vi "Test3-v3-copy1.vi"() -> ()   [LabVIEW 2023]
uses:
  <vilib>/Analysis/8numeric.llb/1D Numeric Integration.vi
  <vilib>/Analysis/NI_AALPro.lvlib
panel:
  out "Is XMotion Done":bool
  out "millisecond timer value":u32
  in  "DoNOT USE":bool
  out "subarray":i32[](array[numeric])
  out "Number areas":i32=1
  out "Gain description":string[](array[string])
  out "ADC description":string[](array[string])
  out "Gain Number":i32[](array[numeric])
  out "activeYPixels":i32=256
  out "activeXPixels":i32=1024
  out "Is YMotion Done":bool
  out "error out":errorcluster
  out "Identification":string
  out "DeviceKey Out":string
  out "Filename":path caption="Filename Out"
  in  "Save?":bool=TRUE caption="Enable"
  in  "CCD Busy 2":bool caption="CCD Busy"
  in  "stop":bool
  in  "Start Scan":bool caption="Acquire"
  out "Acq Time(ms)":u32
  in  "ShutterOpen":bool
  in  "DisplayArea":i32
  in  "numAreas":i32=2
  out "Gain_supplied":i32
  out "ADC_supplied":i32
  out "DataSize":i32
  in  "Number of Areas :":u16=1 min=1 step=1
  in  "Integration time (ms)":i16
  out "ADC Number":i32[](array[numeric])
  out "FirmwareVersion":string="V1.89  CCD_3000"
  out "nbr of components":i32
  out "CCD DeviceName":string[](array[string])
  out "CCD UniqueID":string[](array[string])
  out "Xloop_iter":i32
  out "Yloop_iter":i32
  out "YPos":i32
  out "XPos":i32
  in  "Xtotalsteps":i32
  in  "Xstep_res (BWD)":i32
  in  "Xstep_res (FWD)":i32
  in  "MotorX":i32
  in  "Wait time (ms) in X":u32
  in  "MotorY":i32
  in  "Ystep_res":i32
  in  "Ytotalsteps":i32
  out "max value":i32
  in  "MinZ":dbl
  in  "StopIn":dbl
  in  "StartIn":i32
  out "AreaUnder":dbl format="%0.4f"
  out "Intensity Graph":dbl[][](graph)=[[0.0, 960.0, 940.0, 790.0, 950.0, 1030.0, 970.0, 780.0, 990.0, 1010.0, 980.0, 900.0, 1080.0, 950.0, 890.0, 1020.0, 780.0, 1020.0, 950.0, 1180.0], [800.0, 720.0, 880.0, 950.0, 850.0, 960.0, 940.0, 970.0, 830.0, 1050.0, 1140.0, 870.0, 1000.0, 1340.0, 860.0, 1760.0, 980.0, 1900.0, 1120.0, 1650.0], [770.0, 1000.0, 1080.0, 820.0, 880.0, 880.0, 1170.0, 900.0, 750.0, 1110.0, 950.0, 820.0, 780.0, 1510.0, 710.0, 3630.0, 770.0, 4530.0, 1060.0, 4960.0], [570.0, 1040.0, 990.0, 1300.0, 770.0, 940.0, 940.0, 920.0, 1010.0, 920.0, 1030.0, 1170.0, 670.0, 3990.0, 1270.0, 7770.0, 1780.0, 10190.0, 1940.0, 10320.0], [700.0, 2170.0, 720.0, 1070.0, 920.0, 1100.0, 1070.0, 1240.0, 1090.0, 1090.0, 780.0, 2330.0, 1100.0, 9500.0, 2570.0, 13250.0, 3430.0, 18370.0, 4920.0, 15420.0], [1150.0, 4050.0, 870.0, 1990.0, 990.0, 2300.0, 890.0, 2100.0, 890.0, 2030.0, 850.0, 5530.0, 1660.0, 16900.0, 6920.0, 20860.0, 8010.0, 26820.0, 11920.0, 24090.0], [2410.0, 7690.0, 1380.0, 5680.0, 950.0, 5660.0, 1150.0, 6030.0, 1120.0, 5990.0, 1100.0, 13320.0, 4680.0, 23310.0, 12680.0, 30260.0, 15460.0, 37490.0, 20040.0, 32360.0], [3730.0, 11670.0, 3470.0, 10700.0, 2160.0, 11620.0, 2650.0, 13450.0, 1960.0, 16280.0, 3330.0, 24280.0, 9750.0, 29590.0, 19490.0, 39280.0, 25460.0, 44560.0, 28710.0, 38240.0], [5820.0, 13930.0, 7980.0, 15370.0, 5380.0, 18180.0, 6410.0, 22810.0, 6360.0, 28160.0, 9770.0, 34440.0, 18410.0, 42010.0, 27930.0, 47640.0, 36930.0, 51850.0, 36620.0, 38310.0], [10910.0, 18840.0, 11150.0, 20990.0, 10890.0, 24120.0, 12390.0, 32770.0, 15080.0, 36680.0, 20580.0, 46100.0, 28750.0, 52000.0, 34670.0, 57560.0, 43850.0, 55160.0, 43260.0, 39980.0], [15940.0, 18620.0, 14810.0, 27550.0, 16710.0, 32360.0, 19800.0, 43300.0, 25930.0, 49500.0, 33140.0, 57890.0, 36190.0, 59830.0, 45190.0, 66030.0, 50740.0, 62090.0, 48710.0, 40450.0], [18210.0, 21400.0, 20610.0, 32540.0, 22470.0, 41180.0, 26870.0, 55110.0, 36190.0, 59600.0, 45000.0, 71170.0, 49620.0, 77020.0, 54950.0, 77120.0, 60070.0, 65320.0, 47310.0, 41610.0], [19980.0, 27630.0, 24900.0, 39620.0, 30920.0, 51640.0, 41210.0, 64930.0, 48560.0, 75980.0, 58830.0, 80180.0, 62620.0, 87370.0, 65050.0, 89380.0, 67340.0, 71060.0, 52720.0, 42330.0], [22060.0, 37480.0, 29730.0, 46150.0, 36490.0, 61910.0, 51530.0, 75500.0, 57820.0, 89350.0, 70600.0, 94390.0, 78340.0, 96990.0, 80350.0, 100080.0, 79370.0, 79130.0, 55810.0, 45520.0], [30290.0, 47190.0, 34090.0, 53020.0, 45160.0, 73900.0, 63850.0, 88890.0, 70560.0, 101120.0, 83090.0, 103760.0, 86430.0, 106600.0, 95730.0, 104970.0, 86060.0, 78120.0, 60830.0, 48710.0], [38810.0, 59500.0, 41970.0, 66520.0, 54310.0, 87210.0, 76860.0, 101460.0, 84910.0, 110370.0, 96060.0, 118150.0, 97970.0, 118660.0, 105500.0, 102890.0, 92680.0, 80660.0, 66370.0, 49220.0], [44290.0, 65130.0, 55290.0, 74890.0, 65450.0, 93890.0, 85000.0, 113550.0, 95920.0, 123970.0, 110280.0, 127190.0, 107900.0, 124790.0, 109070.0, 100530.0, 93780.0, 73700.0, 66770.0, 49400.0], [55930.0, 72390.0, 63110.0, 87710.0, 79530.0, 109270.0, 102450.0, 128690.0, 113170.0, 131910.0, 117470.0, 139240.0, 122700.0, 128430.0, 115300.0, 94570.0, 90710.0, 67040.0, 64120.0, 46810.0], [68310.0, 81060.0, 70150.0, 94040.0, 87080.0, 115930.0, 110550.0, 136550.0, 122470.0, 143100.0, 130550.0, 141520.0, 133000.0, 121900.0, 118010.0, 88120.0, 91940.0, 60980.0, 61360.0, 41230.0], [76260.0, 81810.0, 83610.0, 90390.0, 95690.0, 107610.0, 122620.0, 130470.0, 133680.0, 139910.0, 142260.0, 148030.0, 139440.0, 133350.0, 117890.0, 103760.0, 83410.0, 75650.0, 56860.0, 51030.0]]
  out "Data":i32[][](graph)
  out "XY Graph":cluster{"X":dbl[], "Y":dbl[]}[](graph)
  out "result":dbl format="%0.4f"
  out "areas :":i32[][](array[numeric])=[[1], [1], [1], [1440], [1032], [1], [1032]]
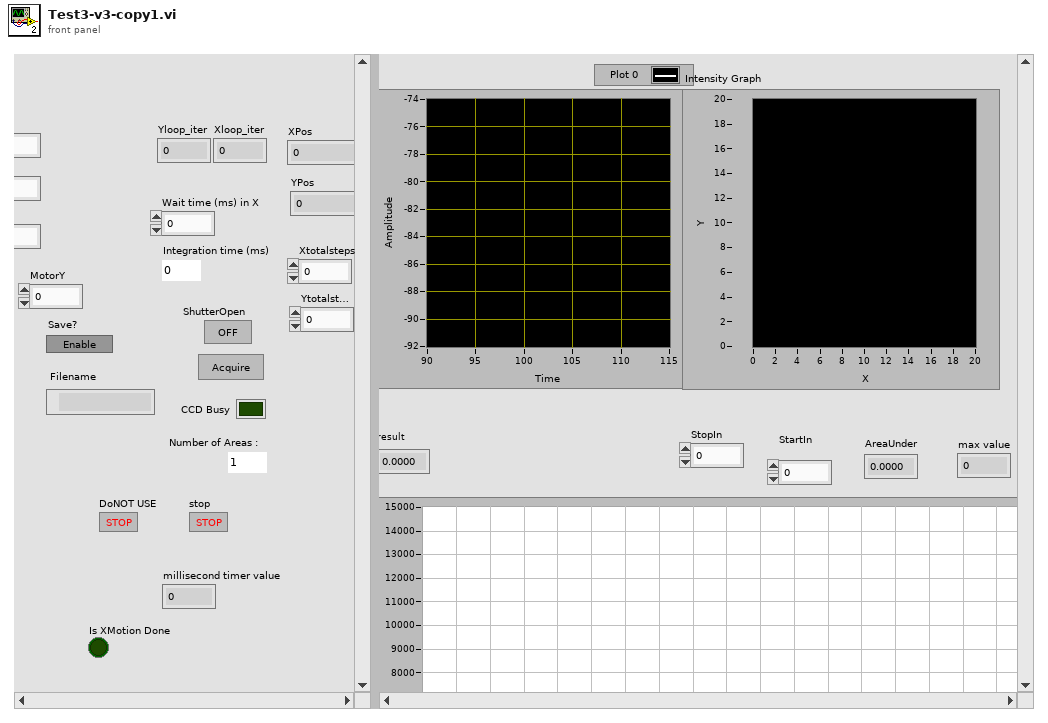
[diagram p1: front panel]
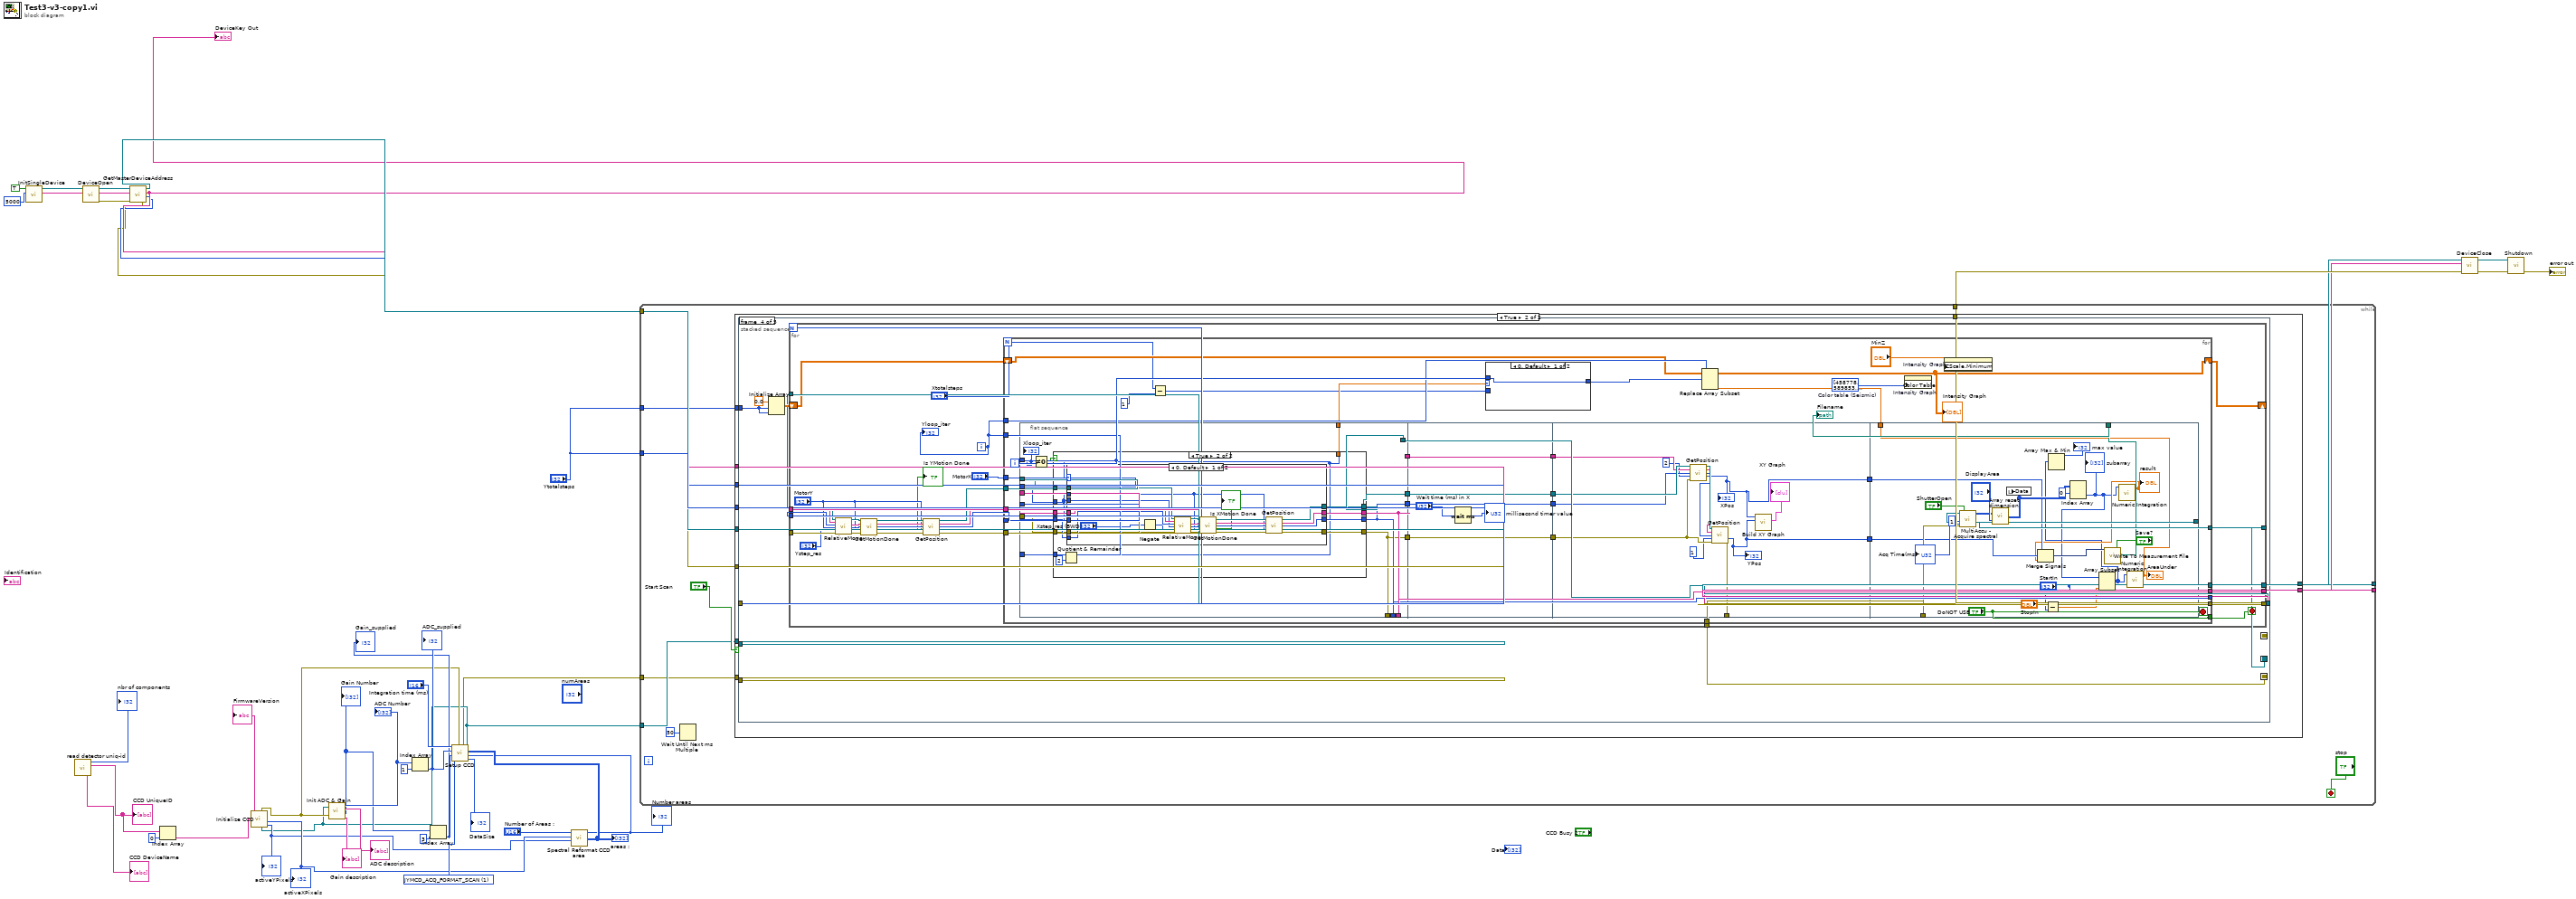
[diagram p0: block diagram]
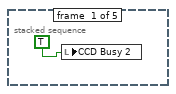
[diagram p3: hidden frame]
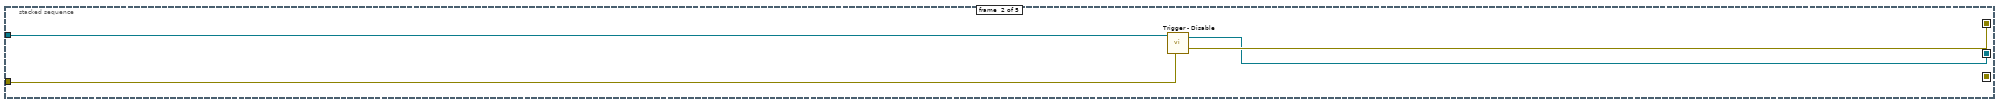
[diagram p4: hidden frame]
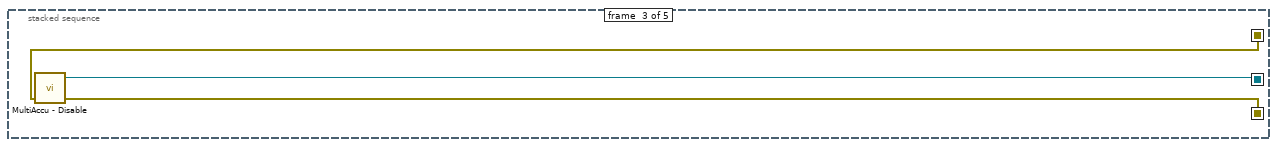
[diagram p5: hidden frame]
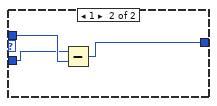
[diagram p6: hidden frame]
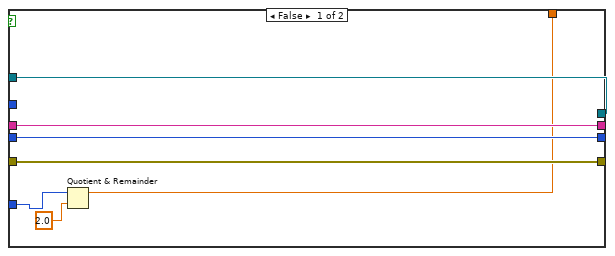
[diagram p7: hidden frame]
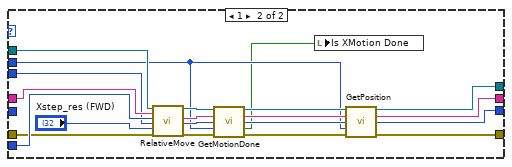
[diagram p8: hidden frame]
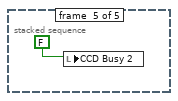
[diagram p9: hidden frame]
diagram:
  w19 = 1 items=["JYMCD_ACQ_FORMAT_IMAGE", "JYMCD_ACQ_FORMAT_SCAN"] ("Acquisition type")
  n1 = call "InitSingleDevice.vi"("msecDelayForDiscovery"=5000, "logging"=TRUE) -> ("DeviceKey Out"=w38:string, "CmdLib Out"=w39:refnum<k24>)  [unwired: 3 in, 1 out]
  n2 = call "read detector uniq-id.vi"() -> ("nbr of components"=→"nbr of components":i32, "UniqueID"=w32:string[], "DeviceName"=→"CCD DeviceName":string[])  [unwired: 3 in, 1 out]
  "CCD UniqueID" <- w32
  n3 = call "DeviceOpen.vi"("DeviceKey In"=w38, "CmdLib In"=w39) -> ("error out"=w42:errorcluster, "DeviceKey Out"=w41:string, "CmdLib Out"=w40:refnum<k24>)  [unwired: 3 in]
  n4 = call "GetMasterDeviceAddress.vi"("error in (no error)"=w42, "DeviceKey In"=w41, "CmdLib In"=w40) -> ("error out"=w5:errorcluster, "Device Address"=w6:i32, "DeviceKey Out"=w7:string, "CmdLib Out"=w8:refnum<k24>)  [unwired: 1 in]
  "DeviceKey Out" <- w7
  n5 = Index Array(array=w32, index=0) -> (element=w30:string)
  n6 = call "Initialize CCD.vi"("Unique id:"=w30) -> ("activeYPixels"=w16:i32, "JYCCDLib.IJYCCDReqd"=w10:refnum<k7>, "activeXPixels"=w17:i32, "sortie d'erreur"=w18:errorcluster, "FirmwareVersion"=→"FirmwareVersion":string)  [unwired: 2 in, 1 out]
  "activeXPixels" <- w17
  "activeYPixels" <- w16
  n7 = call "Init ADC & Gain.vi"("JYCCDLib.IJYCCDReqd"=w10, "input error"=w18) -> ("ADC Number"=w25:i32[], "ADC description"=→"ADC description":string[], "Gain Number"=w22:i32[], "Gain description"=→"Gain description":string[])
  "ADC Number" <- w25
  "Gain Number" <- w22
  n8 = Index Array(array=w25, index=1) -> (element=w23:i32)
  "ADC_supplied" <- w23
  n9 = Index Array(array=w22, index=3) -> (element=w20:i32)
  "Gain_supplied" <- w20
  n10 = call "Spectral Reformat CCD area.vi"("Y Pixels:"=w16, "X Pixels:"=w17, "numAreas"="Number of Areas :") -> ("areas :"=w15:i32[][], "Number areas"=w12:i32)  [unwired: 2 in]
  "areas :" <- w15
  "Number areas" <- w12
  n11 = call "Setup CCD.vi"("numAreas"=w12, "areas :"=w15, "JYCCDLib.IJYCCDReqd"=w10, "entrée d'erreur (pas d'erreur)"=w18, "Acquisition type"=w19, "Gain"=w20, "Select ADC"=w23, "Integration time(ms)"="Integration time (ms)") -> ("DataSize"=→"DataSize":i32, "sortie d'erreur"=w9:errorcluster)
  n12 = while {
    tunnel: w10 -> [w56]
    tunnel: w9 -> [w55]
    tunnel: "Ytotalsteps" -> [w54]
    tunnel: w8 -> [w53]
    tunnel: w7 -> [w52]
    tunnel: w6 -> [w51]
    tunnel: w5 -> [w50]
    tunnel: [w49] -> w4
    tunnel: [w48] -> w3
    tunnel: [w47] -> w2
    tunnel: "Ytotalsteps" -> [w46]
    stop <- "stop" stop-if-true
    n13 = case shown="True" "Start Scan" {
      tunnel: w56 -> [_ w71]
      tunnel: w55 -> [_ w70]
      tunnel: w54 -> [_ w69]
      tunnel: w53 -> [w59 w68]
      tunnel: w52 -> [w58 w67]
      tunnel: w51 -> [_ w66]
      tunnel: w50 -> [w60 w65]
      tunnel: [w60 w64] -> w49
      tunnel: [w58 w63] -> w48
      tunnel: [w59 w62] -> w47
      tunnel: w46 -> [_ w61]
      frame False {
      }
      frame True {
        n14 = stacked-sequence {
          seq-local: [_ w74 _ _ _] -> [_ _ w78 _ _]
          seq-local: [_ w73 _ _ _] -> [_ _ w79 w83 _]
          seq-local: [_ _ w77 _ _] -> [_ _ _ w84 _]
          tunnel: w71 -> [_ w76 _ _ _]
          tunnel: w70 -> [_ w75 _ _ _]
          tunnel: w69 -> [_ _ _ w92 _]
          tunnel: w68 -> [_ _ _ w91 _]
          tunnel: w67 -> [_ _ _ w90 _]
          tunnel: w66 -> [_ _ _ w89 _]
          tunnel: w65 -> [_ _ _ w88 _]
          tunnel: [_ _ _ w87 _] -> w64
          tunnel: [_ _ _ w86 _] -> w63
          tunnel: [_ _ _ w85 _] -> w62
          tunnel: w61 -> [_ _ _ w82 _]
          frame #0 {
            n15 = local write "CCD Busy 2"(TRUE) -> ()
          }
          frame #1 {
            n16 = call "Trigger - Disable.vi"("Error In"=w75, "JYCCDLib.IJYCCDReqd"=w76) -> ("Error Out"=w74:errorcluster, "JYCCDLib.IJYCCDReqd"=w73:refnum<k7>)  [unwired: 4 in]
          }
          frame #2 {
            n17 = call "MultiAccu - Disable.vi"("Error In"=w78, "JYCCDLib.IJYCCDReqd"=w79) -> ("Error Out"=w77:errorcluster)  [unwired: 2 in, 1 out]
          }
          frame #3 {
            n18 = Initialize Array(0.0 ("element"), w82, w82) -> (w80:dbl[][])
            n19 = for {
              N: w92 -> [_]
              tunnel: w91 -> [w114]
              tunnel: w90 -> [w113]
              tunnel: w89 -> [w112]
              tunnel: w88 -> [w111]
              tunnel: [w103] -> w87
              tunnel: [w102] -> w86
              tunnel: [w101] -> w85
              tunnel: w84 -> [w99]
              tunnel: w83 -> [w98]
              shift-right: [w95] -> _
              shift-left: w80 -> [w96]
              i -> [w94]
              stop <- w93 stop-if-true
              n20 = call "RelativeMove.vi"("CmdLib In"=w114, "DeviceKey In"=w113, "Device Address In"=w112, "Motor"="MotorY", "Relative Steps"="Ystep_res", "error in (no error)"=w111) -> ("CmdLib Out"=w118:refnum<k24>, "DeviceKey Out"=w117:string, "Device Address Out"=w116:i32, "error out"=w115:errorcluster)  [unwired: 10 in]
              n21 = call "GetMotionDone.vi"("CmdLib In"=w118, "DeviceKey In"=w117, "Device Address In"=w116, "Motor"="MotorY", "error in (no error)"=w115) -> ("CmdLib Out"=w120:refnum<k24>, "DeviceKey Out"=w119:string, "Device Address Out"=w122:i32, "Is Motion Done"=→"Is YMotion Done":bool, "error out"=w121:errorcluster)  [unwired: 6 in]
              n22 = call "GetPosition.vi"("CmdLib In"=w120, "DeviceKey In"=w119, "Device Address In"=w122, "Motor"="MotorY", "error in (no error)"=w121) -> ("CmdLib Out"=w108:refnum<k24>, "DeviceKey Out"=w107:string, "Device Address Out"=w106:i32, "error out"=w104:errorcluster)  [unwired: 6 in, 1 out]
              n23 = for {
                N: "Xtotalsteps" -> [w138]
                tunnel: w108 -> [w158]
                tunnel: w107 -> [w157]
                tunnel: w106 -> [w156]
                tunnel: "MotorX" -> [w123]
                tunnel: w104 -> [w155]
                tunnel: [w151] -> w103
                tunnel: [w154] -> w102
                tunnel: [w152] -> w101
                tunnel: [w153] -> _
                tunnel: w99 -> [w150]
                tunnel: w98 -> [w149]
                tunnel: w94 -> [w144]
                shift-right: [w142] -> w95
                shift-left: w96 -> [w143]
                tunnel: w94 -> [w141]
                tunnel: ["DoNOT USE"] -> w93
                i -> [w145]
                stop <- "DoNOT USE" stop-if-true
                w135 = u32[] [458778, 589853, 655393, 720933, 852008, 917548, 983087, 1114163, 1179703, 1310778, 1376318, 1441858, 1507397, 1572937, 1572940, 1638480, 1638484, 1704023, 1704027, 1769567, 1769570, 1769574, 1769577, 1835117, 1835121, 1835124, 1835128, 1835132, 1769599, 1769603, 1769606, 1769610, 1704078, 1704081, 1638549, 1638553, 1573020, 1573024, 1507491, 1441959, 1441963, 1376430, 1310898, 1245366, 1179834, 1114307, 1048775, 983243, 917711, 786644, 721116, 655584, 524516, 458984, 327917, 196853, 197113, 66045, 511, 1023, 264703, 528383, 792063, 792063, 1121279, 1384959, 1648639, 1912063, 2241279, 2504703, 2768383, 3031807, 3361023, 3624447, 3887871, 4151295, 4480511, 4743935, 5007359, 5270783, 5533951, 5862911, 6126335, 6389759, 6652927, 6981887, 7245055, 7508479, 7771647, 8100351, 8363775, 8626943, 8890111, 9218815, 9481983, 9745151, 10008063, 10336767, 10599935, 10863103, 11126015, 11454719, 11717631, 11980799, 12243711, 12572159, 12835071, 13098239, 13361151, 13689599, 13952511, 14215167, 14478079, 14806527, 15069439, 15332095, 15595007, 15923199, 16186111, 16448511, 16776958, 16776443, 16775671, 16775155, 16774384, 16773868, 16773096, 16772325, 16771553, 16770781, 16770010, 16769238, 16768466, 16767694, 16766923, 16766151, 16765379, 16764608, 16763580, 16762808, 16762037, 16761009, 16760237, 16759210, 16758438, 16757410, 16756382, 16755611, 16754583, 16753555, 16752528, 16751500, 16750728, 16749701, 16748673, 16747389, 16746362, 16745334, 16744306, 16743278, 16741995, 16740967, 16739939, 16738656, 16737628, 16736344, 16735061, 16734033, 16732749, 16731466, 16730438, 16729154, 16727870, 16726862, 16725835, 16724808, 16724037, 16723010, 16721984, 16721213, 16720186, 16719159, 16718389, 16717362, 16716335, 16715308, 16714538, 16713511, 16712484, 16711714, 16580642, 16580642, 16449570, 16318499, 16187427, 15859747, 15728675, 15597603, 15466531, 15269923, 15007779, 14876708, 14680100, 14549028, 14417956, 14090276, 13959204, 13828132, 13565988, 13369380, 13238308, 13041700, 12845092, 12714020, 12517412, 12320804, 12189731, 11993123, 11796515, 11665443, 11468835, 11272227, 11141155, 10944547, 10747938, 10616866, 10420258, 10223650, 10092578, 9895969, 9699361, 9568289, 9371680, 9175072, 9044000, 8847392, 8650783, 8519711, 8323103, 8126494, 7995422, 7798813, 7602205, 7471133, 7274524, 7077916, 6946843, 6750235, 6553626, 6422554, 6225945, 6029337, 5898264, 5701656, 5505047]  # Color table (Seismic)
                n24 = flat-sequence {
                  tunnel: w158 -> [w175]
                  tunnel: w157 -> [w174]
                  tunnel: w156 -> [w173]
                  tunnel: w123 -> [w172]
                  tunnel: w155 -> [w171]
                  tunnel: [w167] -> _
                  tunnel: [w169] -> w154
                  tunnel: [w168] -> w153
                  tunnel: [w170] -> w152
                  tunnel: [w170] -> w131
                  tunnel: [w169] -> w129
                  tunnel: [w168] -> w127
                  tunnel: [w167] -> w125
                  tunnel: w145 -> [w165]
                  tunnel: w141 -> [w164]
                  tunnel: [w163] -> w140
                  tunnel: w131 -> [w241]
                  tunnel: [w241] -> w130
                  tunnel: w129 -> [w240]
                  tunnel: [w240] -> w128
                  tunnel: w127 -> [w239]
                  tunnel: [w239] -> w126
                  tunnel: w125 -> [w238]
                  tunnel: [w238] -> w124
                  tunnel: w130 -> [w254]
                  tunnel: w128 -> [w253]
                  tunnel: w126 -> [w252]
                  tunnel: w124 -> [w250]
                  tunnel: [w244] -> w151
                  tunnel: [w243] -> w147
                  tunnel: [w242] -> w146
                  tunnel: w150 -> [w272]
                  tunnel: w149 -> [w270]
                  tunnel: [w266] -> w148
                  tunnel: w147 -> [w264]
                  tunnel: w146 -> [w263]
                  tunnel: [w255] -> w132
                  frame #0 {
                    n25 = Not Equal To 0?(x=w165) -> (x != 0?=w166:bool)
                    n26 = case shown="True" w166 {
                      tunnel: w175 -> [w182 w194]
                      tunnel: w174 -> [w181 w193]
                      tunnel: w173 -> [w180 w192]
                      tunnel: w172 -> [_ w186]
                      tunnel: w171 -> [w179 w191]
                      tunnel: [w179 w190] -> w167
                      tunnel: [w181 w189] -> w169
                      tunnel: [w180 w188] -> w168
                      tunnel: [w182 w187] -> w170
                      tunnel: w164 -> [w178 w185]
                      tunnel: [w177 w184] -> w163
                      frame False {
                        n27 = Quotient & Remainder(x=w178, y=2.0) -> (x-y*floor(x/y)=w177:dbl)  [unwired: 1 out]
                      }
                      frame True {
                        n28 = Quotient & Remainder(x=w185, y=2) -> (x-y*floor(x/y)=w184:i32)  [unwired: 1 out]
                        n29 = case shown="0, Default" w184 {
                          tunnel: w194 -> [w207 w228]
                          tunnel: w193 -> [w206 w227]
                          tunnel: w192 -> [w205 w226]
                          tunnel: w186 -> [w195 w225]
                          tunnel: w186 -> [w201 w219]
                          tunnel: w191 -> [w204 w222]
                          tunnel: [w200 w221] -> w190
                          tunnel: [w197 w220] -> w189
                          tunnel: [w199 w218] -> w188
                          tunnel: [w198 w217] -> w187
                          tunnel: w186 -> [_ _]
                          frame 0, Default {
                            n30 = Negate(x="Xstep_res (BWD)") -> (-x=w202:i32)
                            n31 = call "RelativeMove.vi"("CmdLib In"=w207, "DeviceKey In"=w206, "Device Address In"=w205, "Motor"=w195, "Relative Steps"=w202, "error in (no error)"=w204) -> ("CmdLib Out"=w214:refnum<k24>, "DeviceKey Out"=w215:string, "Device Address Out"=w209:i32, "error out"=w208:errorcluster)  [unwired: 10 in]
                            n32 = call "GetMotionDone.vi"("CmdLib In"=w214, "DeviceKey In"=w215, "Device Address In"=w209, "Motor"=w201, "error in (no error)"=w208) -> ("CmdLib Out"=w211:refnum<k24>, "DeviceKey Out"=w210:string, "Device Address Out"=w213:i32, "Is Motion Done"=→"Is XMotion Done":bool, "error out"=w212:errorcluster)  [unwired: 6 in]
                            n33 = call "GetPosition.vi"("CmdLib In"=w211, "DeviceKey In"=w210, "Device Address In"=w213, "Motor"=w201, "error in (no error)"=w212) -> ("CmdLib Out"=w198:refnum<k24>, "DeviceKey Out"=w197:string, "Device Address Out"=w199:i32, "error out"=w200:errorcluster)  [unwired: 6 in, 1 out]
                          }
                          frame 1 {
                            n34 = call "RelativeMove.vi"("CmdLib In"=w228, "DeviceKey In"=w227, "Device Address In"=w226, "Motor"=w225, "Relative Steps"="Xstep_res (FWD)", "error in (no error)"=w222) -> ("CmdLib Out"=w224:refnum<k24>, "DeviceKey Out"=w223:string, "Device Address Out"=w233:i32, "error out"=w234:errorcluster)  [unwired: 10 in]
                            n35 = call "GetMotionDone.vi"("CmdLib In"=w224, "DeviceKey In"=w223, "Device Address In"=w233, "Motor"=w219, "error in (no error)"=w234) -> ("CmdLib Out"=w231:refnum<k24>, "DeviceKey Out"=w232:string, "Device Address Out"=w229:i32, "Is Motion Done"=w216:bool, "error out"=w230:errorcluster)  [unwired: 6 in]
                            n36 = local write "Is XMotion Done"(w216) -> ()
                            n37 = call "GetPosition.vi"("CmdLib In"=w231, "DeviceKey In"=w232, "Device Address In"=w229, "Motor"=w219, "error in (no error)"=w230) -> ("CmdLib Out"=w217:refnum<k24>, "DeviceKey Out"=w220:string, "Device Address Out"=w218:i32, "error out"=w221:errorcluster)  [unwired: 6 in, 1 out]
                          }
                        }
                      }
                    }
                    "Xloop_iter" <- w165
                  }
                  frame #1 {
                    n38 = Wait (ms)(milliseconds to wait="Wait time (ms) in X") -> (millisecond timer value=→"millisecond timer value":u32)
                  }
                  frame #2 {
                    n39 = call "GetPosition.vi"("CmdLib In"=w254, "DeviceKey In"=w253, "Device Address In"=w252, "Motor"=2, "error in (no error)"=w250) -> ("CmdLib Out"=w249:refnum<k24>, "DeviceKey Out"=w248:string, "Device Address Out"=w247:i32, "Position"=w242:i32)  [unwired: 6 in, 1 out]
                    "XPos" <- w242
                    n40 = call "GetPosition.vi"("CmdLib In"=w249, "DeviceKey In"=w248, "Device Address In"=w247, "Motor"=1, "error in (no error)"=w250) -> ("Position"=w243:i32, "error out"=w244:errorcluster)  [unwired: 6 in, 3 out]
                    "YPos" <- w243
                    n41 = call "Build XY Graph"("Y Input"=w243, "X Input"=w242) -> ("XY Graph"=→"XY Graph":cluster{"X":dbl[], "Y":dbl[]}[])  [unwired: 8 in, 1 out]
                  }
                  frame #3 {
                    n42 = call "MultiAccu - Acquire spectral.vi"("error in"=w272, "Accumulations:"=u16 1, "ShutterOpen"="ShutterOpen", "JYCCDLib.IJYCCDReqd"=w270) -> ("Acq Time(ms)"=→"Acq Time(ms)":u32, "Array Out"=w275:i32[][][])  [unwired: 1 out]
                    n43 = call "Array reset dimension.vi"("Area Number"="DisplayArea", "Array In"=w275) -> ("Array Out"=w269:i32[][])
                    n44 = local write "Data"(w269) -> ()
                    n45 = Subtract(x="StopIn", y="StartIn") -> (x-y=w261:dbl)
                    n46 = Index Array(array=w269, index (row)=0) -> (element=w258:i32[])  [unwired: 1 in]
                    "subarray" <- w258
                    n47 = Array Subset(array=w258, index="StartIn", length=w261) -> (w257:i32[])
                    n48 = Array Max & Min(array=w257) -> (max value=→"max value":i32)  [unwired: 3 out]
                    n49 = call-poly <vilib>:"Numeric Integration.vi"("Input Array"=w258) -> ("result"=w262:dbl)  [unwired: 2 in, 1 out]
                    "result" <- w262
                    n50 = Merge Signals(w263, w264, w262) -> (w265:dynamicdata)
                    n51 = call "Write To Measurement File"("Signals"=w265, "Enable"="Save?") -> ("Filename Out"=w266:path)  [unwired: 15 in, 2 out]
                    n52 = call-poly <vilib>:"Numeric Integration.vi"("Input Array"=w257) -> ("result"=w255:dbl)  [unwired: 2 in, 1 out]
                    "AreaUnder" <- w255
                  }
                }
                n53 = Subtract(x=w138, y=1) -> (x-y=w136:i32)
                n54 = case shown="0, Default" w140 {
                  tunnel: w145 -> [w159 w161]
                  tunnel: [w159 w162] -> w139
                  tunnel: w136 -> [_ w160]
                  frame 0, Default {
                  }
                  frame 1 {
                    n55 = Subtract(x=w160, y=w161) -> (x-y=w162:i32)
                  }
                }
                n56 = Replace Array Subset(array=w143, new element=w132, index (row)=w139, index (col)=w144) -> (w142:dbl[][])
                "Intensity Graph" <- w142
                n57 = property on="Intensity Graph" class="IntGraph (strict)"("Color Table"=w135) -> ()  [unwired: 2 in, 2 out]
                n58 = property on="Intensity Graph" class="IntGraph (strict)"("ZScale.Minimum"="MinZ") -> ()  [unwired: 2 in, 2 out]
                "Filename" <- w148
              }
              "Yloop_iter" <- w94
            }
          }
          frame #4 {
            n59 = local write "CCD Busy 2"(FALSE) -> ()
          }
        }
      }
    }
  }
  n60 = Wait Until Next ms Multiple(millisecond multiple=u32 50 ("n millisecondes")) -> ()  [unwired: 1 out]
  n61 = call "DeviceClose.vi"("error in (no error)"=w4, "DeviceKey In"=w3, "CmdLib In"=w2) -> ("error out"=w35:errorcluster, "CmdLib Out"=w36:refnum<k24>)  [unwired: 2 in, 1 out]
  n62 = call "Shutdown.vi"("error in (no error)"=w35, "CmdLib In"=w36) -> ("error out"=→"error out":errorcluster)  [unwired: 4 in, 1 out]
